vi "Measure.vi"(0 "B&K Precision 9120 series in":refnum<class "B&K Precision 9120 series.lvclass">, 5 "error in (no error)":errorcluster) -> (14 "B&K Precision 9120 series out":refnum<class "B&K Precision 9120 series.lvclass">, 15 "Voltage":dbl, 16 "Current":dbl, 17 "CV":bool, 18 "CC":bool, 19 "error out":errorcluster)   [LabVIEW 2014, in "B&K Precision 9120 series.lvclass"]
uses:
  B&K Precision 9120 series.lvclass
  B&K Precision 9120 series.lvclass/B&K Precision 9120 series.ctl
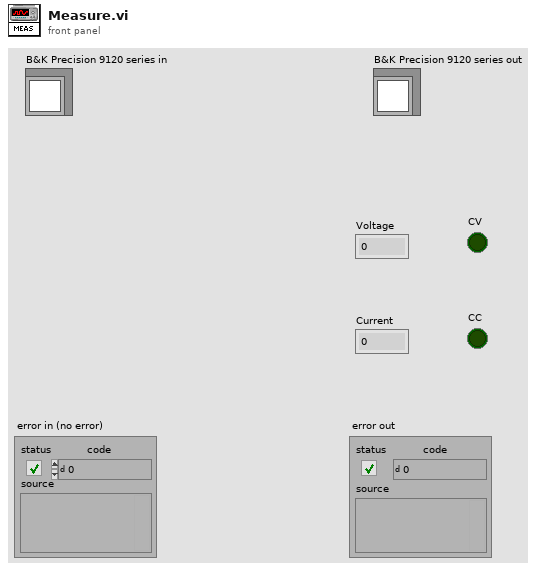
[diagram p1: front panel]
types:
  T1 = typedef "B&K Precision 9120 series.lvclass/Serial_Config.ctl" = cluster{"Baud":u32, "Flow Ctl":u16, "COM port":refnum<visa-resource-name>, "Parity":u16}
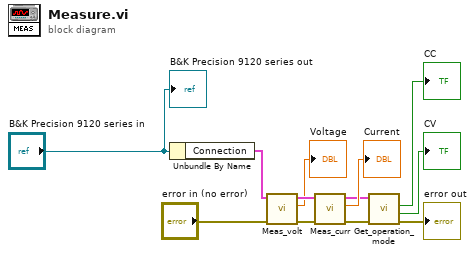
[diagram p0: block diagram]
diagram:
  n1 = Unbundle By Name("B&K Precision 9120 series in") -> ("Connection"=w11:T1)
  n2 = call "Meas_volt.vi"("error in (no error)"="error in (no error)", "Connection in"=w11) -> ("error out"=w12:errorcluster, "Voltage"=→"Voltage":dbl, "Connection out"=w10:T1)  [unwired: 7 in]
  n3 = call "Meas_curr.vi"("error in (no error)"=w12, "Connection in"=w10) -> ("error out"=w6:errorcluster, "Current"=→"Current":dbl, "Connection out"=w7:T1)  [unwired: 7 in]
  n4 = call "Get_operation_mode.vi"("error in (no error)"=w6, "Connection in"=w7) -> ("error out"=→"error out":errorcluster, "CV"=→"CV":bool, "CC"=→"CC":bool)  [unwired: 6 in, 1 out]
  "B&K Precision 9120 series out" <- "B&K Precision 9120 series in"
